vi "SQLite Get Fields Info.vi"(8 "error in":errorcluster, 10 "Table Name":string="test", 11 "SQLite Connection":refnum<class "Connection.lvclass">) -> (0 "error out":errorcluster, 2 "Fields Info":T1[](array[typedef]), 3 "Dup SQLite Connection":refnum<class "Connection.lvclass">)   [LabVIEW 2021, in "EDT SQLite+.lvlib"]
uses:
  EDT SQLite+.lvlib
  SQLite Field Info.ctl
  SQLite Data Type.ctl
  <vilib>/drjdpowell/SQLite Library/SQL Connection/Connection.lvclass
  <vilib>/drjdpowell/SQLite Library/SQL Statement/SQL Statement.lvclass/SQL Statement.ctl
  <vilib>/drjdpowell/SQLite Library/SQL Statement/Column I64.vi
  <vilib>/drjdpowell/SQLite Library/SQL Statement/Error Message.vi
  <vilib>/drjdpowell/SQLite Library/SQL Statement/Column String.vi
  <vilib>/drjdpowell/SQLite Library/SQL Statement/Column Variant.vi
  <vilib>/drjdpowell/SQLite Library/SQL Statement/SQL Statement.lvclass
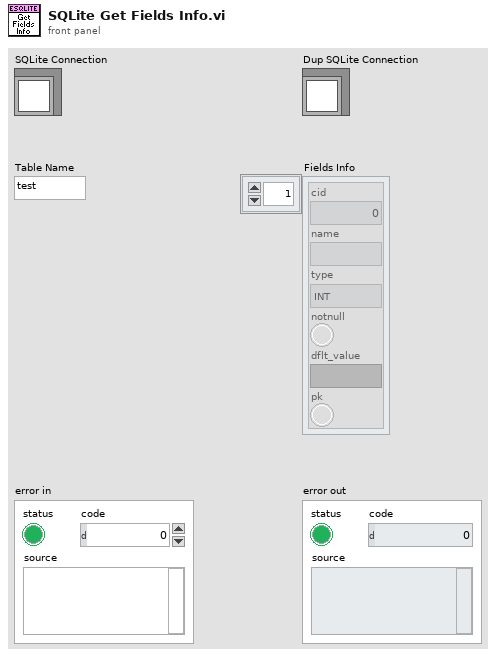
[diagram p1: front panel]
types:
  T1 = typedef "EDT SQLite+.lvlib/SQLite Field Info.ctl" = cluster{"cid":i32, "name":string, "type":T2, "notnull":bool, "dflt_value":variant, "pk":bool}
  T2 = typedef "EDT SQLite+.lvlib/SQLite Data Type.ctl" = enum16{"INT", "INTEGER", "TINYINT", "SMALLINT", "MEDIUMINT", "BIGINT", "UNSIGNED BIG INT", "INT2", "INT8", "CHARACTER", "VARCHAR", "VARYING CHARACTER", "NCHAR", "NATIVE CHARACTER", "NVARCHAR", "TEXT", "CLOB", "BLOB", "no datatype specified", "REAL", "DOUBLE", "DOUBLE PRECISION", "FLOAT", "NUMERIC", "DECIMAL", "BOOLEAN", "DATE", "DATETIME"}
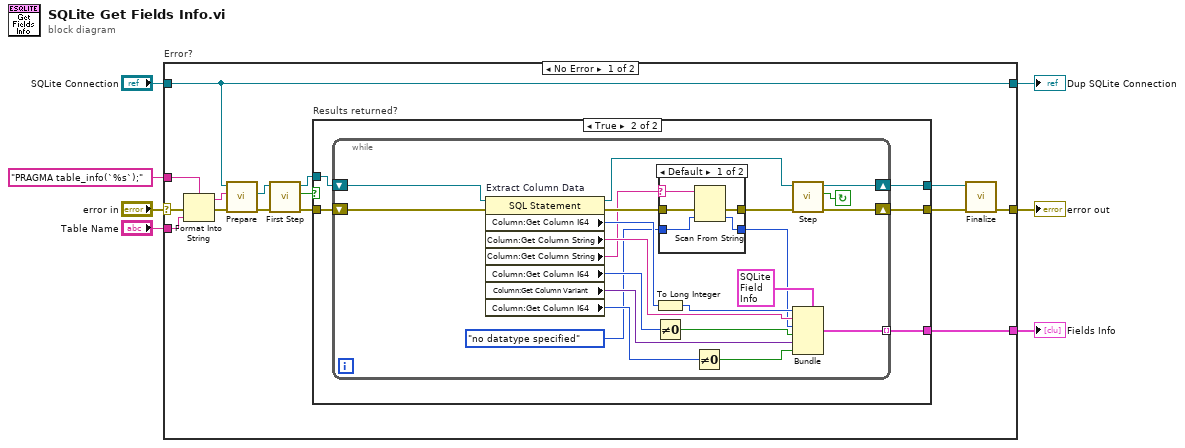
[diagram p0: block diagram]
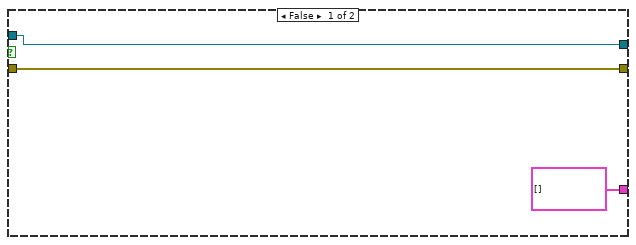
[diagram p2: hidden frame]
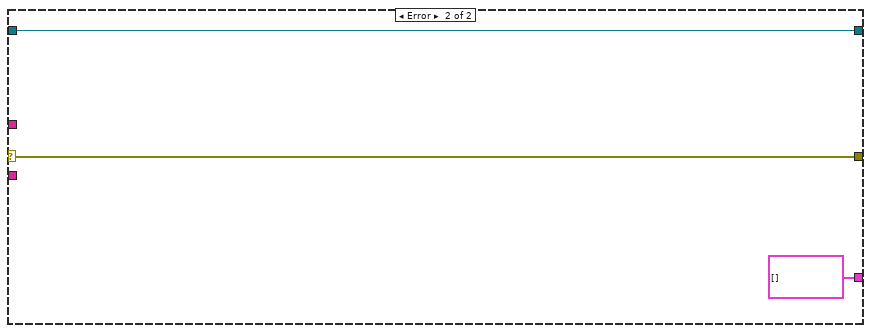
[diagram p4: hidden frame]
diagram:
  n1 = case "Error?" shown="No Error" "error in" {
    selector: "error in" -> [w9 w61]
    tunnel: "Table Name" -> [w19 _]
    tunnel: [w22 T1[] []] -> w3
    tunnel: [w21 w61] -> w5
    tunnel: "PRAGMA table_info(`%s`);" ("SELECT  statement") -> [w20 _]
    tunnel: "SQLite Connection" -> [w10 w59]
    tunnel: [w10 w59] -> w1
    frame No Error {
      n2 = Format Into String(format string=w20, error in=w9, w19) -> (resulting string=w18:string, error out=w8:errorcluster)  [unwired: 1 in]
      n3 = call <vilib>:"Prepare.vi"("error in (no error)"=w8, "SQL"=w18, "SQLite Connection in"=w10) -> ("error out"=w11:errorcluster, "SQL Statement"=w12:refnum<class "SQL Statement.lvclass">)  [unwired: 4 in, 3 out]
      n4 = call <vilib>:"First Step.vi"("error in (no error)"=w11, "SQL Statement in"=w12) -> ("error out"=w14:errorcluster, "Row returned"=w13:bool, "SQL Statement"=w15:refnum<class "SQL Statement.lvclass">)  [unwired: 7 in]
      n5 = case "Results returned?" shown="True" w13 {
        tunnel: [w25 w30] -> w16
        tunnel: [w24 w29] -> w17
        tunnel: w15 -> [w25 w28]
        tunnel: w14 -> [w24 w27]
        tunnel: [T1[] [] w26] -> w22
        frame False {
        }
        frame True {
          n6 = while "For each row..." {
            shift-right: [w50] -> w30
            shift-left: w28 -> [w48]
            shift-right: [w49] -> w29
            shift-left: w27 -> [w47]
            tunnel: [w36] -> w26 mode=indexing
            stop <- w46 continue-if-true
            n7 = property on="Extract Column Data" class="SQL Statement"(reference=w48, error in=w47) -> (reference out=w51:refnum<class "SQL Statement.lvclass">, error out=w33:errorcluster, "Column:Get Column I64"=w45:i64, "Column:Get Column String"=w44:string, "Column:Get Column String"=w31:string, "Column:Get Column I64"=w43:i64, "Column:Get Column Variant"=w42:variant, "Column:Get Column I64"=w41:i64)
            n8 = To Long Integer(number=w45) -> (32bit integer=w37:i32)
            n9 = Not Equal To 0?(x=w43) -> (x != 0?=w39:bool)
            n10 = case shown="Default" w31 {
              selector: w31 -> [w52 _]
              tunnel: SQLite_Data_Type."no datatype specified" ("SQLite Data Type") -> [w56 w57]
              tunnel: [w55 w57] -> w34
              tunnel: w33 -> [w54 w58]
              tunnel: [w53 w58] -> w32
              frame Default {
                n11 = Scan From String(input string=w52, error in=w54, default 1=w56) -> (error out=w53:errorcluster, output 1=w55:T2)  [unwired: 2 in, 2 out]
              }
              frame "\u0000" {
              }
            }
            n12 = Not Equal To 0?(x=w41) -> (x != 0?=w40:bool)
            n13 = call <vilib>:"Step.vi"("error in (no error)"=w32, "SQL Statement in"=w51) -> ("error out"=w49:errorcluster, "Row returned"=w46:bool, "SQL Statement"=w50:refnum<class "SQL Statement.lvclass">)  [unwired: 7 in]
            n14 = Bundle(cluster=T1 {"cid"=0, "name"="", "type"=enum."INT", "notnull"=FALSE, "dflt_value"=variant, "pk"=FALSE} ("column info"), "cid"=w37, "name"=w44, "type"=w34, "notnull"=w39, "dflt_value"=w42, "pk"=w40) -> (w36:T1)
          }
        }
      }
      n15 = call <vilib>:"Finalize.vi"("error in (no error)"=w17, "SQL Statement in"=w16) -> ("error out"=w21:errorcluster)  [unwired: 9 in]
    }
    frame Error {
    }
  }
  "error out" <- w5
  "Fields Info" <- w3
  "Dup SQLite Connection" <- w1
